vi "set default exposure time.vi"(8 "error in (no error)":errorcluster, 11 "Thorcam in":refnum<class "Thorcam.lvclass">) -> (0 "error out":errorcluster, 1 "exposure time":dbl[unit], 3 "Thorcam out":refnum<class "Thorcam.lvclass">)   [LabVIEW 2012, in "Thorcam.lvclass"]
uses:
  Thorcam.lvclass
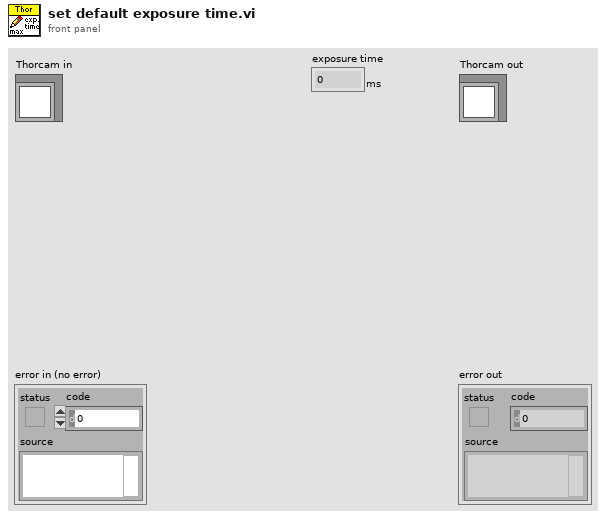
[diagram p1: front panel]
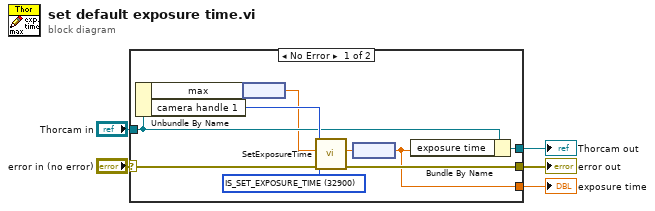
[diagram p0: block diagram]
diagram:
  n1 = case shown="No Error" "error in (no error)" {
    selector: "error in (no error)" -> [w14 w17]
    tunnel: [w13 w17] -> w4
    tunnel: [w10 w16] -> w2
    tunnel: "Thorcam in" -> [w11 w16]
    tunnel: [w8 _] -> w1
    frame No Error {
      w12 = u16 32900 items=["IS_SET_EXPOSURE_TIME"=32900, "IS_GET_EXPOSURE_TIME"=32768, "IS_GET_DEFAULT_EXPOSURE"=32769] ("Mode")
      n2 = Unbundle By Name(w11) -> ("max"=w7:dbl[unit], "camera handle 1"=w15:u32)
      n3 = node(w7) -> (w6:dbl)
      n4 = call <instrlib>:"SetExposureTime.vi"("error in"=w14, "Mode"=w12, "Exposure Time"=w6, "Camera Handle In"=w15) -> ("error out"=w13:errorcluster, "new exposure time"=w9:dbl)  [unwired: 5 in, 1 out]
      n5 = node(w9) -> (w8:dbl[unit])
      n6 = Bundle By Name(cluster=w11, "exposure time"=w8) -> (w10:refnum<class "Thorcam.lvclass">)
    }
    frame Error {
    }
  }
  "error out" <- w4
  "Thorcam out" <- w2
  "exposure time" <- w1
